vi "Safe Move.vi"(9 "Directions in":i32[](array[numeric]), 10 "Action in":T1, 11 "Fortress In":refnum<class "Fortress.lvclass">) -> (0 "Accepted?":bool, 1 "Direction":T2, 2 "Action out":T1, 3 "Fortress Out":refnum<class "Fortress.lvclass">)   [LabVIEW 2017, in "Fortress.lvclass"]
uses:
  Fortress.lvclass
  Type Defs/Action Enum.ctl
  Type Defs/Direction Enum.ctl
  Fortress.lvclass/Fortress.ctl
  Common/Common.lvlib
  Type Defs/SB Type Defs.lvlib
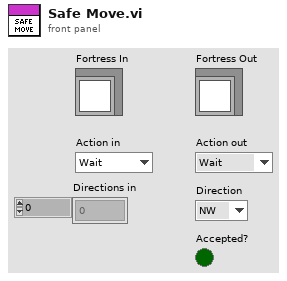
[diagram p1: front panel]
types:
  T1 = typedef "SB Type Defs.lvlib/Action Enum.ctl" = enum16{"Wait", "Move", "Attack", "Replicate"}
  T2 = typedef "SB Type Defs.lvlib/Direction Enum.ctl" = enum16{"NW", "N", "NE", "E", "SE", "S", "SW", "W"}
  T3 = typedef "Common.lvlib/Position.ctl" = cluster{"Column":i32, "Row":i32}
  T4 = typedef "Common.lvlib/Map DVR.ctl" = refnum<data-value>
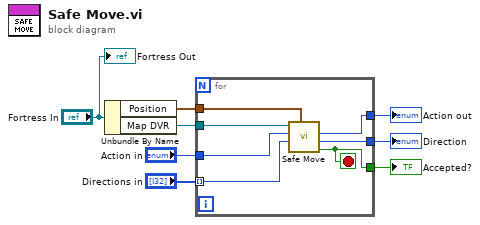
[diagram p0: block diagram]
diagram:
  n1 = Unbundle By Name("Fortress In") -> ("Position"=w6:T3, "Map DVR"=w1:T4)
  n2 = for {
    tunnel: "Directions in" -> [w15] mode=indexing
    tunnel: w6 -> [w13]
    tunnel: [w12] -> w5
    tunnel: [w10] -> w2
    tunnel: "Action in" -> [w14]
    tunnel: [w11] -> w4
    tunnel: w1 -> [w9]
    stop <- w10 stop-if-true
    n3 = call "Safe Move.vi"("Position in"=w13, "Direction in"=w15, "Desired Action"=w14, "Map DVR"=w9) -> ("Accepted?"=w10:bool, "Direction"=w12:T2, "Action"=w11:T1)  [unwired: 4 in, 1 out]
  }
  "Direction" <- w5
  "Action out" <- w4
  "Accepted?" <- w2
  "Fortress Out" <- "Fortress In"
